vi "add_exclusion_to_graph.vi"(0 "Rot(rad)":dbl=3.6441621315637374 step=0.1 format="%.2f", 3 "acrmin/pulse":dbl=5.28e-05 format="%.4e", 4 "CentreTel Y":i32=70736 min=0 max=1000000 step=1000, 5 "PulseyCentre":i32=41801 min=0 max=1000000 step=1000, 6 "CentreTel X":i32=647041 min=0 max=1000000 step=1000, 7 "2er couple":string, 8 "1er couple":string, 9 "PulsexCentre":i32=641444 min=0 max=1000000 step=1000) -> (1 "Cavenas":cluster{dbl[], dbl[]}, 2 "line one":cluster{dbl[], dbl[]})   [LabVIEW 2010]
panel:
  out "XY Graph":cluster{dbl[], dbl[]}(graph)
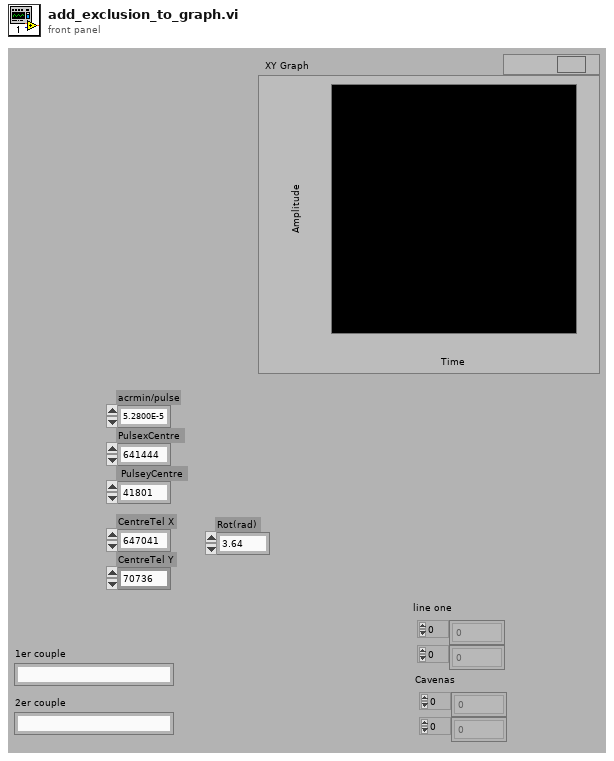
[diagram p1: front panel]
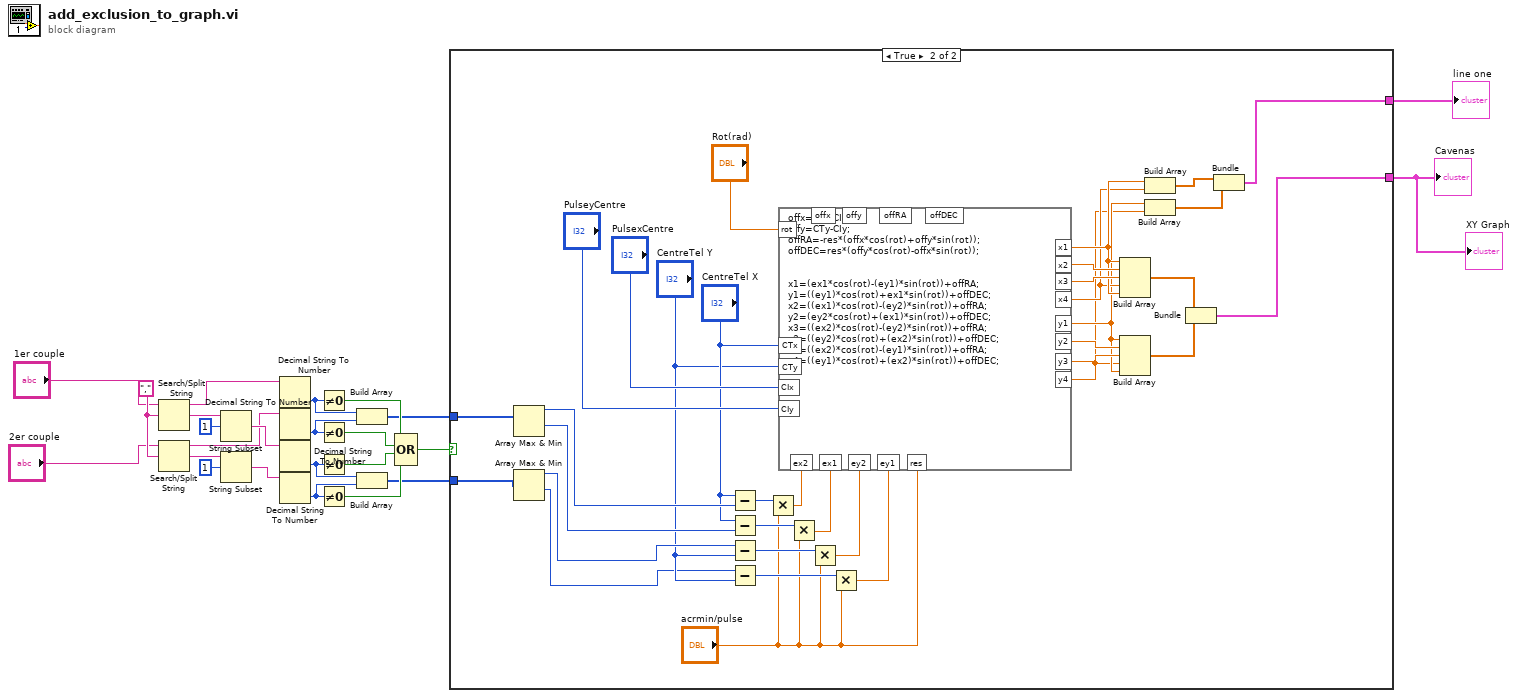
[diagram p0: block diagram]
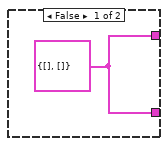
[diagram p2: hidden frame]
diagram:
  w24 = "," ("search string/char (-)")
  n1 = Search/Split String(string="1er couple", search string/char (-)=w24) -> (substring before match=w21:string, match + rest of string=w22:string)  [unwired: 1 in, 1 out]
  n2 = Search/Split String(string="2er couple", search string/char (-)=w24) -> (substring before match=w3:string, match + rest of string=w23:string)  [unwired: 1 in, 1 out]
  n3 = String Subset(string=w22, offset (0)=1) -> (substring=w4:string)  [unwired: 1 in]
  n4 = String Subset(string=w23, offset (0)=1) -> (substring=w20:string)  [unwired: 1 in]
  n5 = Decimal String To Number(string=w21) -> (number=w14:i32)  [unwired: 2 in, 1 out]
  n6 = Decimal String To Number(string=w3) -> (number=w13:i32)  [unwired: 2 in, 1 out]
  n7 = Decimal String To Number(string=w4) -> (number=w12:i32)  [unwired: 2 in, 1 out]
  n8 = Decimal String To Number(string=w20) -> (number=w11:i32)  [unwired: 2 in, 1 out]
  n9 = Not Equal To 0?(x=w14) -> (x != 0?=w15:bool)
  n10 = Not Equal To 0?(x=w13) -> (x != 0?=w19:bool)
  n11 = Not Equal To 0?(x=w12) -> (x != 0?=w18:bool)
  n12 = Not Equal To 0?(x=w11) -> (x != 0?=w17:bool)
  n13 = Build Array(w14, w13) -> (w10:i32[])
  n14 = Build Array(w12, w11) -> (w9:i32[])
  n15 = Compound Arithmetic op=OR(w15, w19, w18, w17) -> (w16:bool)
  n16 = case shown="True" w16 {
    tunnel: w10 -> [_ w46]
    tunnel: w9 -> [_ w47]
    tunnel: [w25 w36] -> w2
    tunnel: [w25 w33] -> w1
    frame False {
      w25 = cluster{dbl[], dbl[]} {[], []}
    }
    frame True {
      n17 = Array Max & Min(array=w46) -> (max value=w50:i32, min value=w48:i32)  [unwired: 2 out]
      n18 = Array Max & Min(array=w47) -> (max value=w28:i32, min value=w26:i32)  [unwired: 2 out]
      n19 = Subtract(x="CentreTel X", y=w50) -> (x-y=w45:i32)
      n20 = Subtract(x="CentreTel X", y=w48) -> (x-y=w44:i32)
      n21 = Subtract(x=w28, y="CentreTel Y") -> (x-y=w43:i32)
      n22 = Subtract(x=w26, y="CentreTel Y") -> (x-y=w42:i32)
      n23 = Multiply(x=w45, y="acrmin/pulse") -> (x*y=w40:dbl)
      n24 = Multiply(x=w44, y="acrmin/pulse") -> (x*y=w39:dbl)
      n25 = Multiply(x=w43, y="acrmin/pulse") -> (x*y=w38:dbl)
      n26 = Multiply(x=w42, y="acrmin/pulse") -> (x*y=w37:dbl)
      n27 = formula code="offx=CTx-CIx;\noffy=CTy-CIy;\noffRA=-res*(offx*cos(rot)+offy*sin(rot));\noffDEC=res*(offy*cos(rot)-offx*sin(rot));\n\n  \nx1=(ex1*cos(rot)-(ey1)*sin(rot))+offRA;\ny1=((ey1)*cos(rot)+ex1*sin(rot))+offDEC;\nx2=((ex1)*cos(rot)-(ey2)*sin(rot))+offRA;\ny2=(ey2*cos(rot)+(ex1)*sin(rot))+offDEC;\nx3=((ex2)*cos(rot)-(ey2)*sin(rot))+offRA;\ny3=((ey2)*cos(rot)+(ex2)*sin(rot))+offDEC;\nx4=((ex2)*cos(rot)-(ey1)*sin(rot))+offRA;\ny4=((ey1)*cos(rot)+(ex2)*sin(rot))+offDEC;"("rot"="Rot(rad)", "CTx"="CentreTel X", "CTy"="CentreTel Y", "CIx"="PulsexCentre", "CIy"="PulseyCentre", "res"="acrmin/pulse", "ex1"=w39, "ex2"=w40, "ey1"=w37, "ey2"=w38) -> ("x1"=w32:dbl, "x2"=w56:dbl, "y1"=w30:dbl, "y2"=w53:dbl, "x3"=w55:dbl, "x4"=w31:dbl, "y3"=w54:dbl, "y4"=w29:dbl)  [unwired: 4 out]
      n28 = Build Array(w32, w56, w55, w31, w32) -> (w52:dbl[])
      n29 = Build Array(w30, w53, w54, w29, w30) -> (w51:dbl[])
      n30 = Build Array(w32, w31) -> (w34:dbl[])
      n31 = Build Array(w30, w29) -> (w35:dbl[])
      n32 = Bundle(w52, w51) -> (w36:cluster{dbl[], dbl[]})  [unwired: 1 in]
      n33 = Bundle(w34, w35) -> (w33:cluster{dbl[], dbl[]})  [unwired: 1 in]
    }
  }
  "Cavenas" <- w2
  "XY Graph" <- w2
  "line one" <- w1
